vi "Avg Image Path.vi"(8 "error in (no error)":errorcluster, 10 "Avg ImagePath":path, 11 "Image Averaging in":refnum<class "Image Averaging.lvclass">) -> (0 "error out":errorcluster, 3 "Image Averaging out":refnum<class "Image Averaging.lvclass">)   [LabVIEW 2022 SP3, in "Image Averaging.lvlib" / "Image Averaging.lvclass"]
uses:
  Image Averaging.lvclass
  Image Averaging.lvclass/Image Averaging.ctl
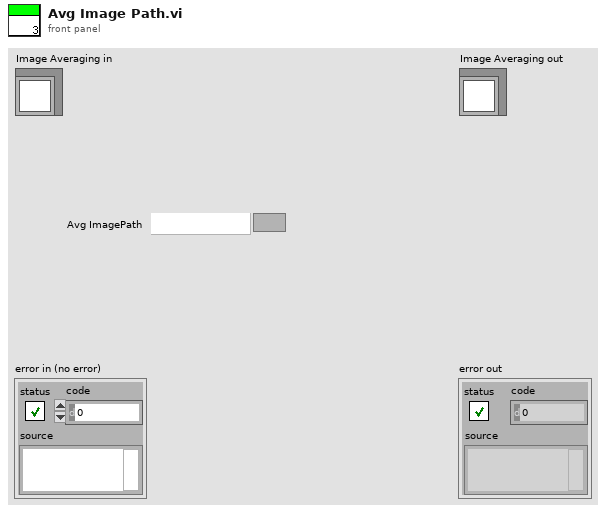
[diagram p1: front panel]
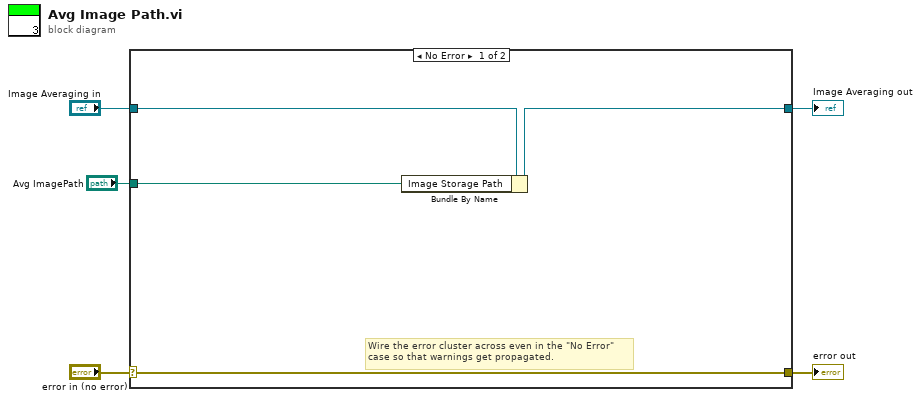
[diagram p0: block diagram]
diagram:
  n1 = case shown="No Error" "error in (no error)" {
    selector: "error in (no error)" -> [w8 w11]
    tunnel: [w8 w11] -> w4
    tunnel: [w7 w10] -> w2
    tunnel: "Image Averaging in" -> [w9 w10]
    tunnel: "Avg ImagePath" -> [w6 _]
    frame No Error {
      # "Wire the error cluster across even in the \"No Error\"\ncase so that warnings get propagated."
      n2 = Bundle By Name(cluster=w9, "Image Storage Path"=w6) -> (w7:refnum<class "Image Averaging.lvclass">)
    }
    frame Error {
    }
  }
  "error out" <- w4
  "Image Averaging out" <- w2
